vi "Stop Core.vi"(10 "final error code":i32, 11 "LoggedActor in":refnum<class "LoggedActor.lvclass">) -> (3 "LoggedActor out":refnum<class "LoggedActor.lvclass">)   [LabVIEW 2019, in "LoggedActor.lvclass"]
doc: "(<B>Filename</B>: Actor Framework.lvlib:Actor.lvclass:Stop Core.vi)\n\nDefines what the actor does before it stops. Use the <B>final error code</B> input to determine whether the actor shut down in response to an error.\n\nBy default, this method does nothing. A descendant class may override it to define behavior, such as shutting down any processes the actor initiated in its override of the Actor Core method."
uses:
  <vilib>/gpm_packages/@cs/Network-interface/Source/Logged Actor/LoggedActor.lvclass
  <vilib>/gpm_packages/@cs/event-logger/Source/Composed Log/Types/Log Level.ctl
  <vilib>/gpm_packages/@cs/Network-interface/Source/Logged Actor/LoggedActor.lvclass/LoggedActor.ctl
  <vilib>/gpm_packages/@cs/event-logger/Source/Composed Log/LoggerReference/LoggerReference.lvclass/LoggerReference.ctl
  <vilib>/gpm_packages/@cs/event-logger/Source/Composed Log/LoggerReference/Log Event.vi
  <vilib>/gpm_packages/@cs/event-logger/Source/Composed Log/LoggerReference/Log.vi
  <vilib>/gpm_packages/@cs/event-logger/Source/Composed Log/LoggerReference/Get Valid Event Time.vi
  <vilib>/gpm_packages/@cs/event-logger/Source/Composed Log/LoggerReference/Remove Stale Logs.vi
  <vilib>/ActorFramework/Actor/Actor.lvclass
  <vilib>/gpm_packages/@cs/event-logger/Source/Composed Log/Composed Log.lvlib
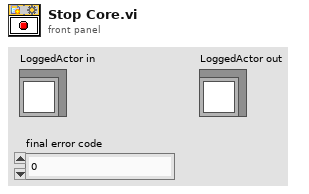
[diagram p1: front panel]
types:
  T1 = typedef "Composed Log.lvlib/Log Level.ctl" = enum16{"Debug", "Info", "Warning", "Error", "Critical"}
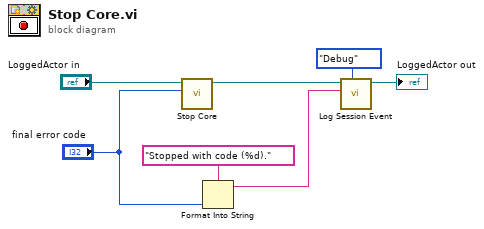
[diagram p0: block diagram]
diagram:
  n1 = call-parent "Stop Core.vi"("final error code"="final error code", "Actor in"="LoggedActor in") -> ("Actor out"=w6:refnum<class "LoggedActor.lvclass">)  [unwired: 9 in]
  n2 = Format Into String(format string="Stopped with code (%d).", "final error code") -> (resulting string=w2:string)  [unwired: 2 in, 1 out]
  n3 = call <vilib>:"Log Session Event.vi"("Event Level"=Log_Level."Debug", "Event Data"=w2, "SessionActor in"=w6) -> ("SessionActor out"=→"LoggedActor out":refnum<class "LoggedActor.lvclass">)  [unwired: 7 in, 1 out]
